vi "CST_Reg_CONFIG1.vi"() -> (0 "CONFIG1":T1={"DAISY_EN"=enum."Multiple Readback Mode", "CLK_EN"=enum."Output Disabled", "DR"=enum."f(MOD) /128"} caption="Configuration Register 1 (CONFIG1)")   [LabVIEW 2010]
uses:
  Controls/Register/TYP_Reg_CONFIG1.ctl
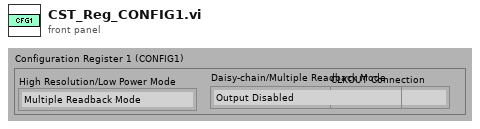
[diagram p1: front panel]
types:
  T1 = typedef "TYP_Reg_CONFIG1.ctl" = cluster{"DAISY_EN":enum16{"Daisy Chain Mode", "Multiple Readback Mode"}, "CLK_EN":enum16{"Output Disabled", "Output Enabled"}, "DR":enum16{"f(MOD) /64", "f(MOD) /128", "f(MOD) /256", "f(MOD) /512", "f(MOD) /1024", "f(MOD) /2048", "f(MOD) /4096"}}
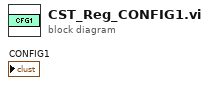
[diagram p0: block diagram]
diagram:
